vi "Space del to num array.vi"(11 "Input in":string) -> (3 "Input out":u64[](array[numeric]))   [LabVIEW 2020, in "Map.lvclass"]
uses:
  Map/Map.lvclass
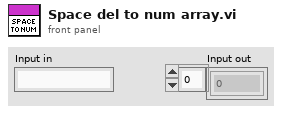
[diagram p1: front panel]
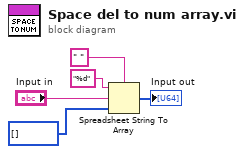
[diagram p0: block diagram]
diagram:
  n1 = Spreadsheet String To Array(delimiter (Tab)=" ", format string="%d", spreadsheet string="Input in", array type (2D Dbl)=u64[] [] ("Input")) -> (array=→"Input out":u64[])
